vi "sync_write.vi"() -> ()   [LabVIEW 2015]
uses:
  dxl_x86_c.lvlib/dxl_x86_c.lvlib
panel:
  out "group_num":i32
  in  "LEN_MX_\nGOAL_POSITION":u16=2
  out "value : MX (knob)\npresent position 2":u16(knob)
  in  "dynamixe2_id":u8=2
  in  "device_name":string="COM8"
  in  "ADDR_MX_\nPRESENT_POSITION":u16=36
  in  "ADDR_MX_\nGOAL_POSITION":u16=30
  in  "ADDR_MX_\nTORQUE_ENABLE":u16=24
  out "protocol_version":dbl=1.0
  out "value : MX (knob)\npresent position 1":u16(knob)
  in  "terminate":bool
  out "port_num":i32
  in  "value : MX (dial)\ngoal position":u16(knob)
  in  "dynamixel1_id":u8=1
  in  "baud_rate":i32=1000000
  # "sync_write.vi\n\nCreated on: 2016. 6. 13\nAuthor: Leon Ryu Woon Jung\n\n*********     Sync Write Example      ********\n\n\nAvailable Dynamixel model on this example : All models using Protocol 1.0\nThis example is designed for using two Dynamixel MX-28, and an USB2DYNAMIXEL.\nTo use another Dynamixel model, such as X series, see their details in E-Manual(support.robotis.com) and edit below variables yourself.\nBe sure that Dynamixel MX properties are already set as %% ID : 1 / Baudnum : 1 (Baudrate : 1000000 [1M])\n\n\n1. Run example by click above \"Run\" button (below \"Edit\" menu).\n2. Drag \"dial\" then you may see the Dynamixel and \"knob\"s rotating\n3. To finish the example, press \"terminate\" button."
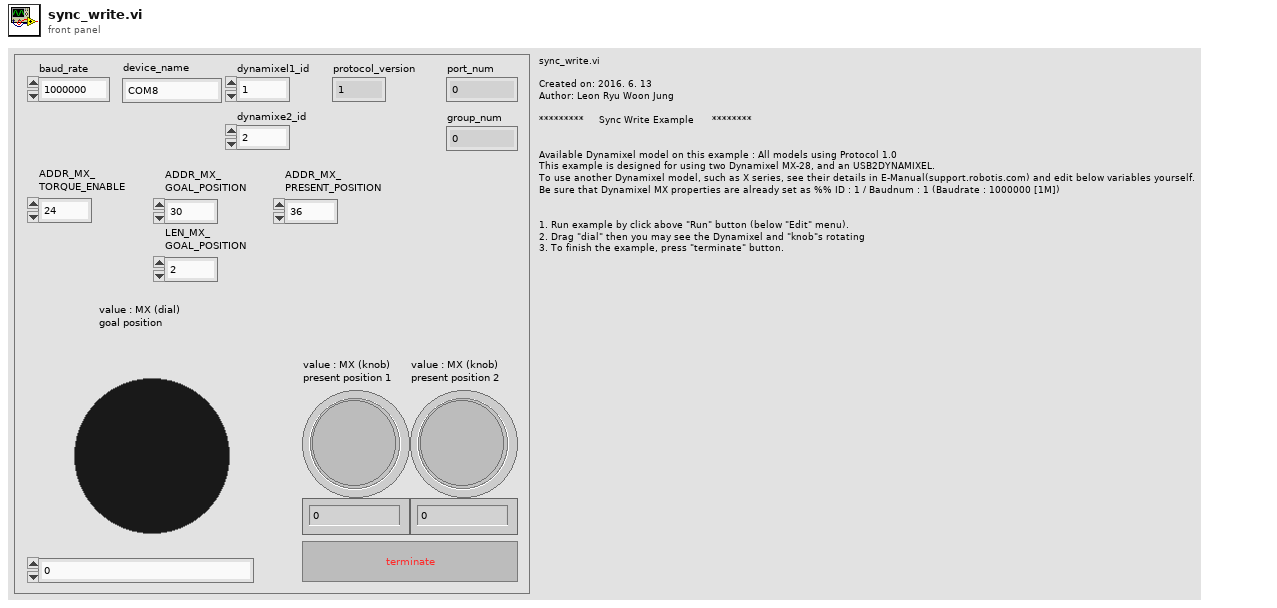
[diagram p1: front panel]
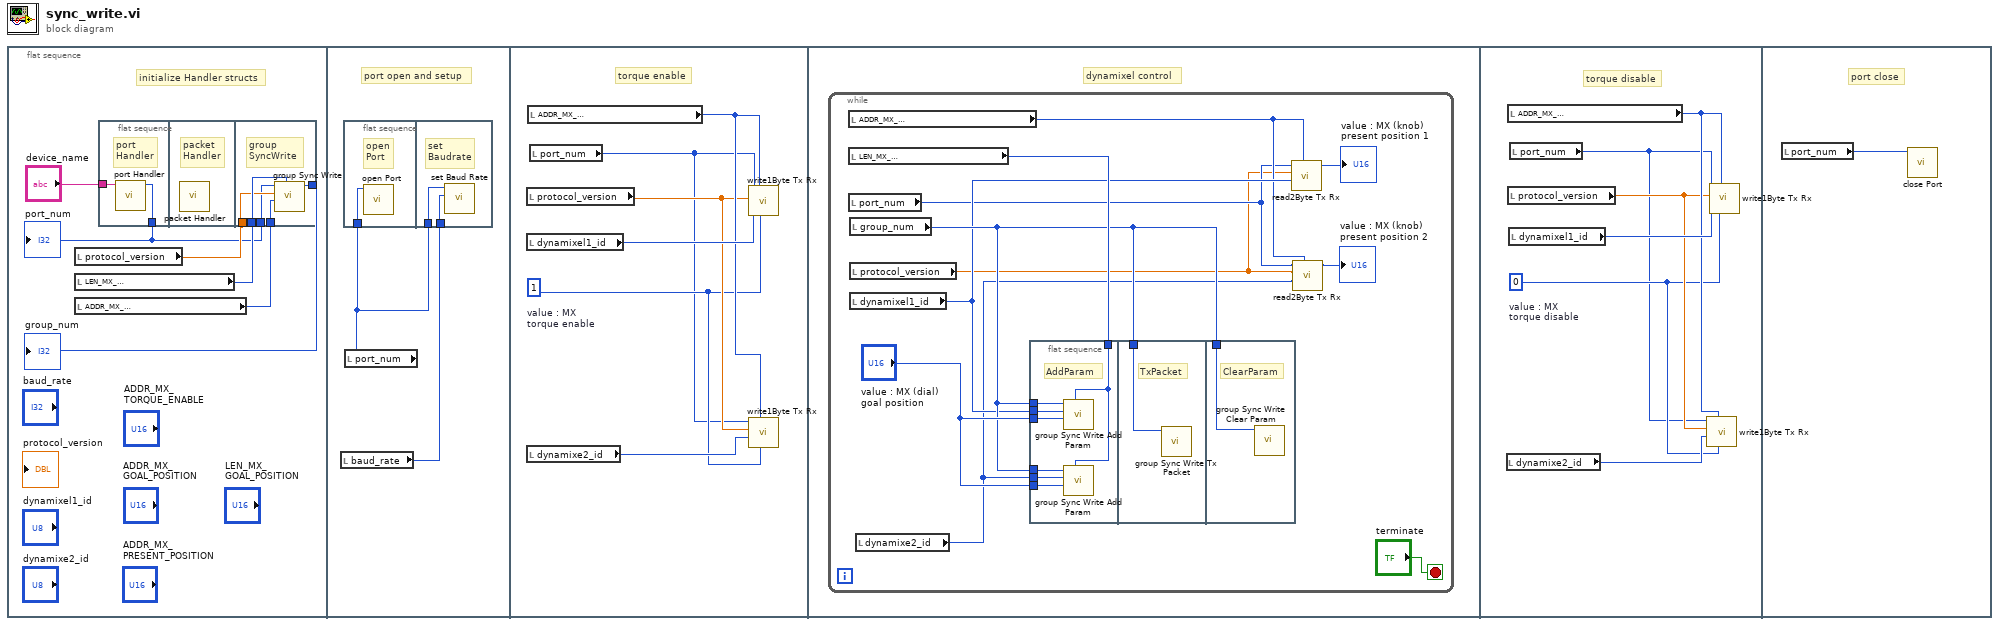
[diagram p0: block diagram]
diagram:
  n1 = flat-sequence {
    frame #0 {
      # "initialize Handler structs"
      n2 = local read "protocol_version"() -> (w3:dbl)
      n3 = local read "LEN_MX_\nGOAL_POSITION"() -> (w5:u16)
      n4 = local read "ADDR_MX_\nGOAL_POSITION"() -> (w4:u16)
      n5 = flat-sequence {
        tunnel: "device_name" -> [w8]
        tunnel: [w7] -> w2
        tunnel: w5 -> [w13]
        tunnel: w4 -> [w12]
        tunnel: w3 -> [w11]
        tunnel: w2 -> [w10]
        tunnel: [w9] -> w1
        frame #0 {
          # "port\nHandler"
          n6 = call "port Handler.vi"("port_name"=w8) -> ("function return"=w7:i32)  [unwired: 10 in]
        }
        frame #1 {
          # "packet\nHandler"
          n7 = call "packet Handler.vi"() -> ()  [unwired: 12 in]
        }
        frame #2 {
          # "group\nSyncWrite"
          n8 = call "group Sync Write.vi"("data_length"=w13, "start_address"=w12, "protocol_version"=w11, "port_num"=w10) -> ("function return"=w9:i32)  [unwired: 7 in]
        }
      }
      "port_num" <- w2
      "group_num" <- w1
    }
    frame #1 {
      # "port open and setup"
      n9 = local read "baud_rate"() -> (w14:i32)
      n10 = flat-sequence {
        tunnel: w15 -> [w16]
        tunnel: w15 -> [w18]
        tunnel: w14 -> [w17]
        frame #0 {
          # "open\nPort"
          n11 = call "open Port.vi"("port_num"=w16) -> ()  [unwired: 10 in, 1 out]
        }
        frame #1 {
          # "set\nBaudrate"
          n12 = call "set Baud Rate.vi"("baudrate"=w17, "port_num"=w18) -> ()  [unwired: 9 in, 1 out]
        }
      }
      n13 = local read "port_num"() -> (w15:i32)
    }
    frame #2 {
      w20 = 1  # value : MX torque enable
      # "torque enable"
      n14 = local read "protocol_version"() -> (w22:dbl)
      n15 = local read "dynamixel1_id"() -> (w24:u8)
      n16 = local read "dynamixe2_id"() -> (w21:u8)
      n17 = local read "ADDR_MX_\nTORQUE_ENABLE"() -> (w23:u16)
      n18 = local read "port_num"() -> (w19:i32)
      n19 = call "write1Byte Tx Rx.vi"("data"=w20, "address"=w23, "id"=w24, "protocol_version"=w22, "port_num"=w19) -> ()  [unwired: 7 in]
      n20 = call "write1Byte Tx Rx.vi"("data"=w20, "address"=w23, "id"=w21, "protocol_version"=w22, "port_num"=w19) -> ()  [unwired: 7 in]
    }
    frame #3 {
      # "dynamixel control"
      n21 = while {
        stop <- "terminate" stop-if-true
        n22 = local read "ADDR_MX_\nPRESENT_POSITION"() -> (w30:u16)
        n23 = local read "LEN_MX_\nGOAL_POSITION"() -> (w34:u16)
        n24 = local read "port_num"() -> (w29:i32)
        n25 = local read "group_num"() -> (w32:i32)
        n26 = local read "protocol_version"() -> (w28:dbl)
        n27 = local read "dynamixel1_id"() -> (w31:u8)
        n28 = local read "dynamixe2_id"() -> (w27:u8)
        n29 = flat-sequence {
          tunnel: w34 -> [w42]
          tunnel: w32 -> [w41]
          tunnel: w32 -> [w40]
          tunnel: w31 -> [w39]
          tunnel: w27 -> [w38]
          tunnel: "value : MX (dial)\ngoal position" -> [w37]
          tunnel: "value : MX (dial)\ngoal position" -> [w36]
          tunnel: w32 -> [w43]
          tunnel: w32 -> [w44]
          frame #0 {
            # "AddParam"
            n30 = call "group Sync Write Add Param.vi"("data_length"=w42, "data"=w36, "id"=w39, "group_num"=w41) -> ()  [unwired: 7 in, 1 out]
            n31 = call "group Sync Write Add Param.vi"("data_length"=w42, "data"=w37, "id"=w38, "group_num"=w40) -> ()  [unwired: 7 in, 1 out]
          }
          frame #1 {
            # "TxPacket"
            n32 = call "group Sync Write Tx Packet.vi"("group_num"=w43) -> ()  [unwired: 11 in]
          }
          frame #2 {
            # "ClearParam"
            n33 = call "group Sync Write Clear Param.vi"("group_num"=w44) -> ()  [unwired: 11 in]
          }
        }
        n34 = call "read2Byte Tx Rx.vi"("address"=w30, "id"=w31, "protocol_version"=w28, "port_num"=w29) -> ("function return"=→"value : MX (knob)\npresent position 1":u16)  [unwired: 7 in]
        n35 = call "read2Byte Tx Rx.vi"("address"=w30, "id"=w27, "protocol_version"=w28, "port_num"=w29) -> ("function return"=→"value : MX (knob)\npresent position 2":u16)  [unwired: 7 in]
      }
    }
    frame #4 {
      w46 = 0  # value : MX torque disable
      # "torque disable"
      n36 = local read "dynamixe2_id"() -> (w47:u8)
      n37 = local read "ADDR_MX_\nTORQUE_ENABLE"() -> (w49:u16)
      n38 = local read "protocol_version"() -> (w48:dbl)
      n39 = local read "dynamixel1_id"() -> (w50:u8)
      n40 = local read "port_num"() -> (w45:i32)
      n41 = call "write1Byte Tx Rx.vi"("data"=w46, "address"=w49, "id"=w47, "protocol_version"=w48, "port_num"=w45) -> ()  [unwired: 7 in]
      n42 = call "write1Byte Tx Rx.vi"("data"=w46, "address"=w49, "id"=w50, "protocol_version"=w48, "port_num"=w45) -> ()  [unwired: 7 in]
    }
    frame #5 {
      # "port close"
      n43 = local read "port_num"() -> (w51:i32)
      n44 = call "close Port.vi"("port_num"=w51) -> ()  [unwired: 11 in]
    }
  }
